vi "PPMSDR - Read lockin vs time_1.0.vi"(8 "stop":bool, 10 "Comments":string="Warmup\nVbg=0V\nVsg: NA\n\n200uV ac\nI+/I-: 2/5 200uVac\nI2+/-: 27/3 200uVac\nV+/V-: 3/27\nV3+/-: 4/28\nVsg: NA\n", 11 "folder name":string="monitor") -> (1 "X1":cluster{"Y":dbl[], "Y":dbl[]}[](graph), 3 "Temp vs Time":cluster{"Y":dbl[], "Y":dbl[]}[](graph), 5 "X4":cluster{"Y":dbl[], "Y":dbl[]}[](graph))   [LabVIEW 2013]
uses:
  <userlib>/Levylab/PPMS VI/Lock-in Globles.vi
  <userlib>/Levylab/PPMS VI/SubVI/ITX_Global.vi
  QDServer/QDServGlobal.vi
  <vilib>/Utility/file.llb/Write To Spreadsheet File (string).vi
panel:
  in  "Tab Control":T1(tab)
  in  "milliseconds to wait":u32=1000
  out "Connected":string="I-:4\nV2+:28\nI+:1\nV1+:2\nV-:3\nV2-:5\n"
  in  "Lockins":i32[](array[numeric])=[0, 1, 2, 3, 4, 5]
  out "Array X":dbl[](array[numeric])=[5.264924893925422e-11, 1.3604655963589375e-10, 5.1217581158894604e-08, 4.031695120308963e-16, -1.3552086788225654e-05, 3.1233416285824434e-11]
  out "Array Y":dbl[](array[numeric])=[-3.141694202030661e-12, -8.008054257042766e-12, -2.1068074715954563e-08, 8.074647968603996e-16, 1.39380477016865e-07, -2.3056960893811664e-13]
  in  "2 Frequencies?":bool
  out "X0":cluster{"Y":dbl[], "Y":dbl[]}[](graph)
  out "X2":cluster{"Y":dbl[], "Y":dbl[]}[](graph)
  out "X3":cluster{"Y":dbl[], "Y":dbl[]}[](graph)
  out "X5":cluster{"Y":dbl[], "Y":dbl[]}[](graph)
  out "R":cluster{"Y":dbl[], "Y":dbl[]}[](graph)
  in  "V1":i32
  in  "Current":i32=1
  in  "V2":i32
  out "B vs Time":cluster{"Y":dbl[], "Y":dbl[]}[](graph)
  out "R vs T":cluster{"Y":dbl[], "Y":dbl[]}[](graph)
  # "0,1,2,3 ect."
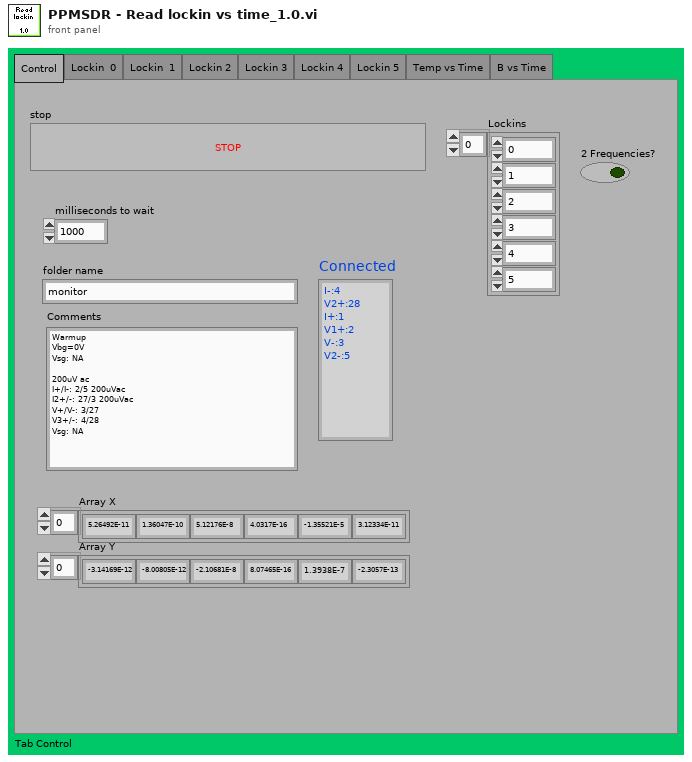
[diagram p1: front panel]
types:
  T1 = enum32{"Control", "Lockin  0", "Lockin  1", "Lockin 2", "Lockin 3", "Lockin 4", "Lockin 5", "Temp vs Time", "B vs Time"}
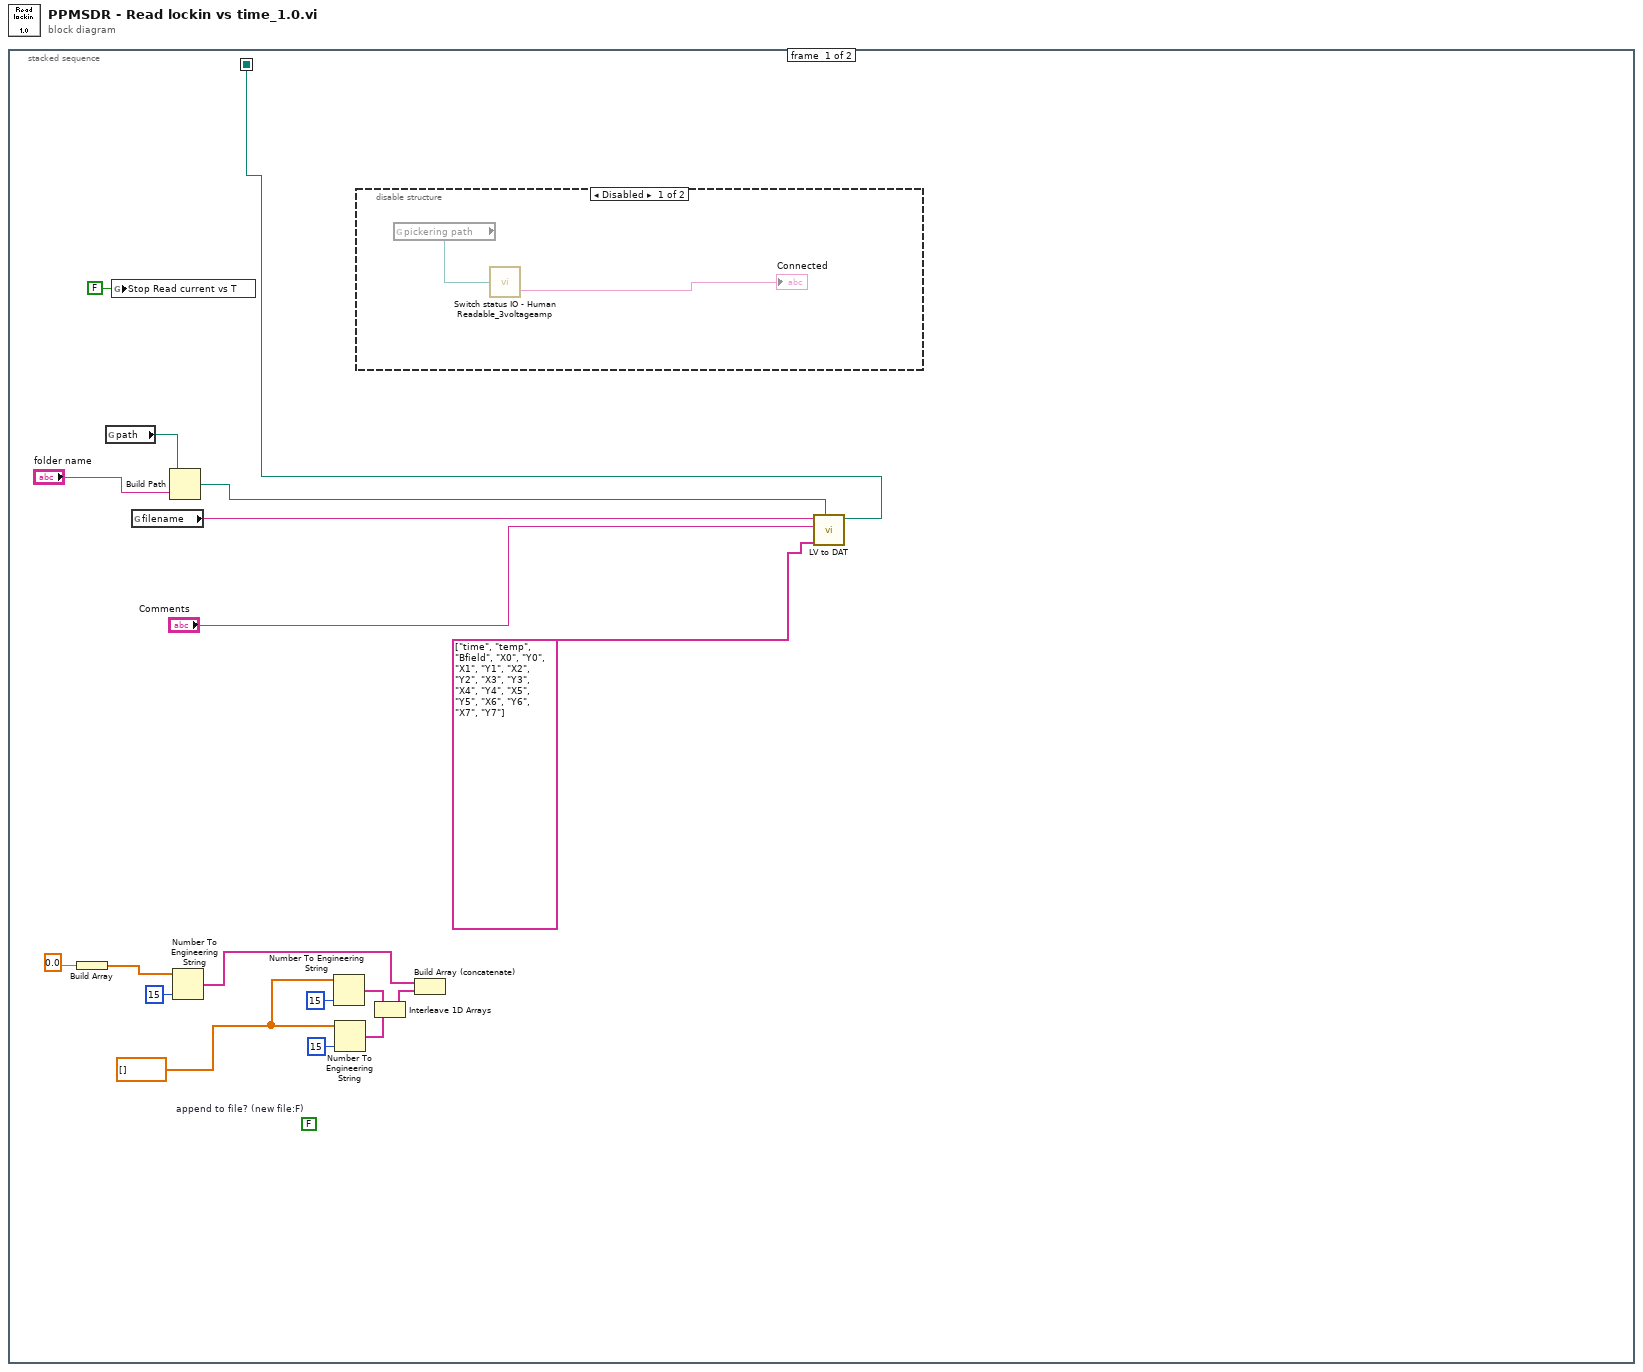
[diagram p0: block diagram]
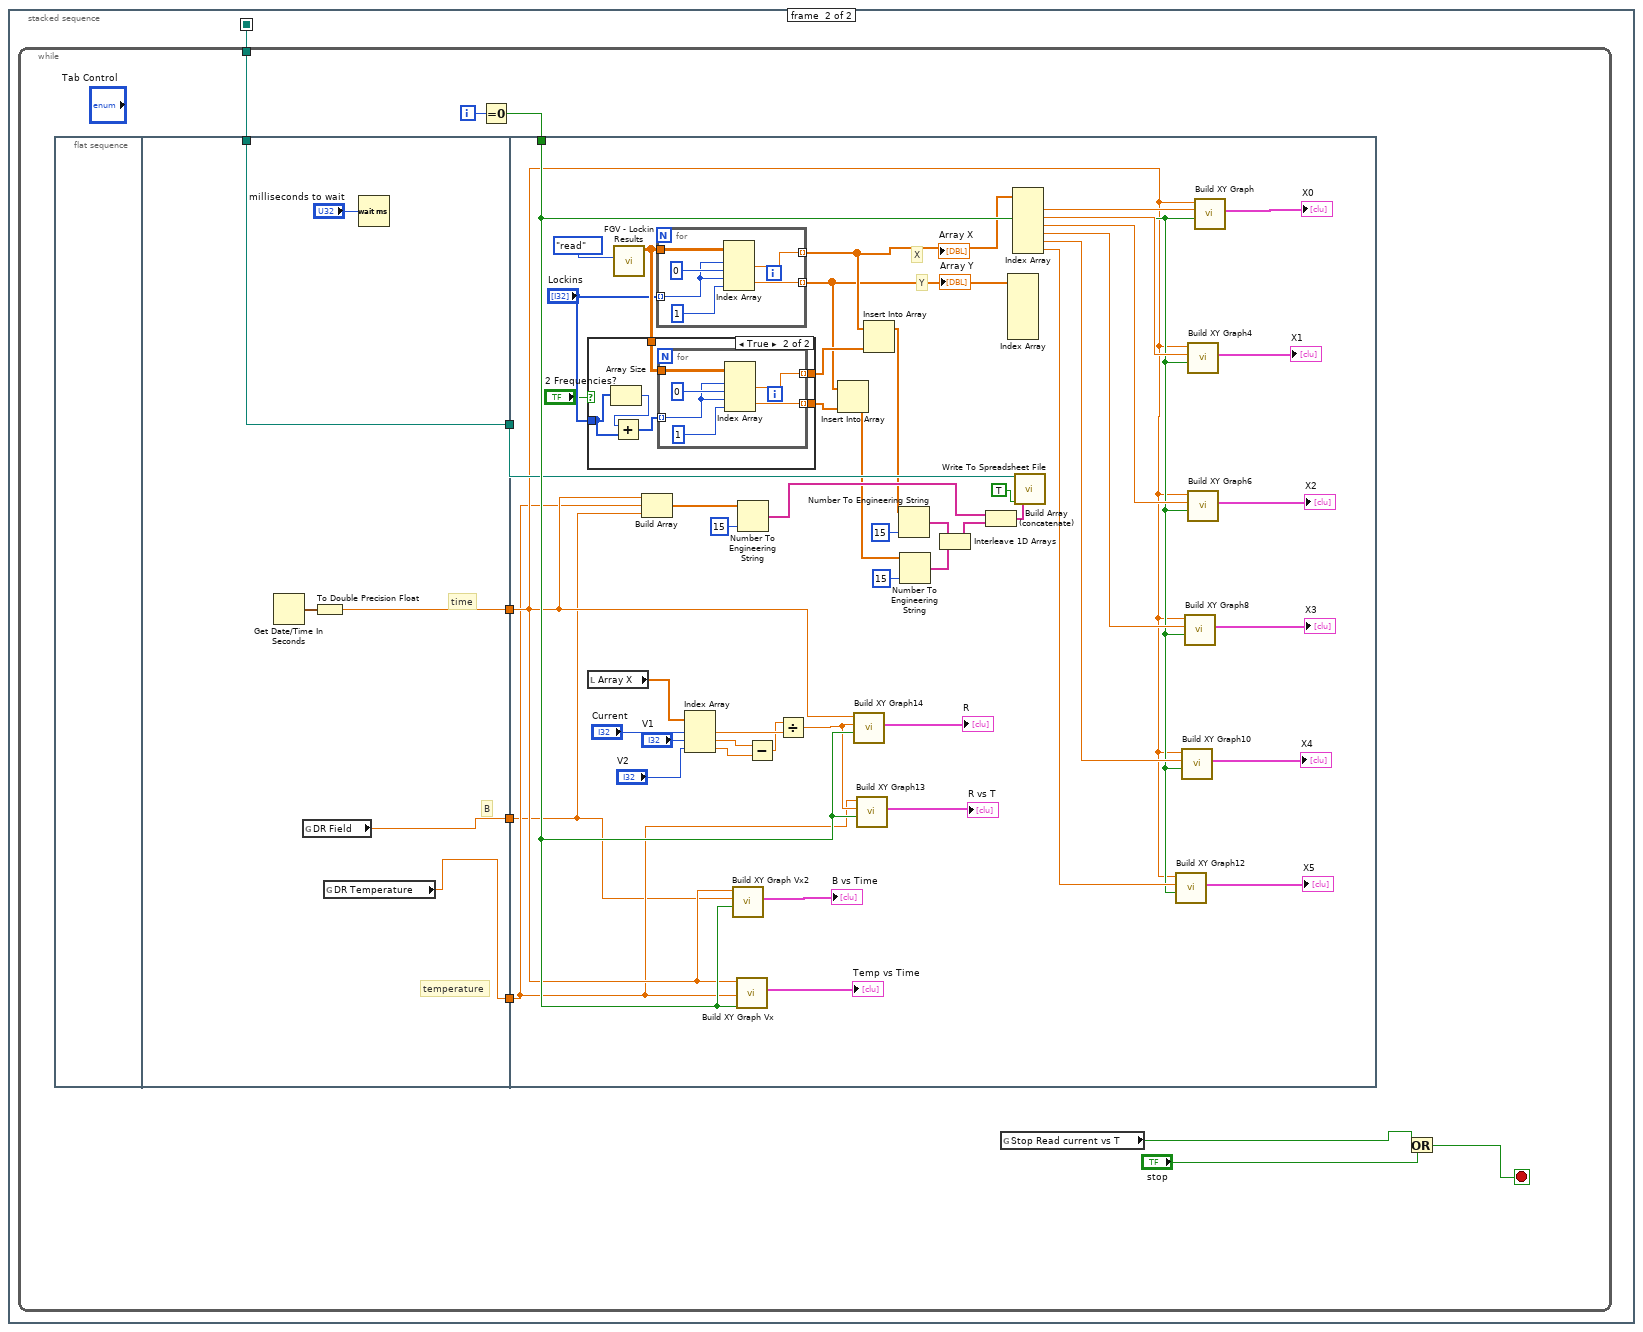
[diagram p3: hidden frame]
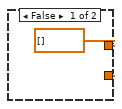
[diagram p4: hidden frame]
diagram:
  n1 = stacked-sequence {
    seq-local: [w1 _] -> [_ w21]
    frame #0 {
      w6 = dbl[] []
      (unwired) FALSE  # append to file? (new file:F)
      n2 = Build Array(0.0) -> (w12:dbl[])
      n3 = global read "ITX_Global.vi" "path"() -> (w17:path)
      n4 = global write "Lock-in Globles.vi" "Stop Read current vs T"(FALSE ("Stop Read current vs T")) -> ()
      n5 = global read "ITX_Global.vi" "filename"() -> (w3:string)
      n6 = Build Path(base path=w17, name or relative path="folder name") -> (appended path=w2:path)
      n7 = Number To Engineering String(2:i16 15 ("precision (6)"), 4:w12) -> (0:w11:string[])  [unwired: 2 out]
      n8 = Number To Engineering String(2:i16 15 ("precision (6)"), 4:w6) -> (0:w10:string[])  [unwired: 2 out]
      n9 = Number To Engineering String(2:i16 15 ("precision (6)"), 4:w6) -> (0:w9:string[])  [unwired: 2 out]
      n10 = disable-structure shown="Disabled" {
        frame Disabled {
          n11 = global read "ITX_Global.vi" "pickering path"() -> (w19:path)
          n12 = call <userlib>:"Switch status IO - Human Readable_3voltageamp.vi"("Switch status"=w19) -> ("String"=→"Connected":string)  [unwired: 3 in]
        }
        frame Enabled {
        }
      }
      n13 = Interleave 1D Arrays(w10, w9) -> (w8:string[])
      n14 = Build Array (concatenate)(w11, w8) -> ()  [unwired: 1 out]
      n15 = call <userlib>:"LV to DAT.vi"("path"=w2, "wavenames (.Vx, etc)"=string[] ["time", "temp", "Bfield", "X0", "Y0", "X1", "Y1", "X2", "Y2", "X3", "Y3", "X4", "Y4", "X5", "Y5", "X6", "Y6", "X7", "Y7"], "Comments"="Comments", "filename"=w3) -> ("new file path (Not A Path if cancelled)"=w1:path)  [unwired: 7 in]
    }
    frame #1 {
      n16 = while {
        tunnel: w21 -> [w24]
        i -> [w31]
        stop <- w25 stop-if-true
        n17 = flat-sequence {
          tunnel: [w35] -> w29
          tunnel: [w32] -> w27
          tunnel: [w33] -> w26
          tunnel: w24 -> [w34]
          tunnel: [w34] -> w23
          tunnel: w30 -> [w66]
          tunnel: w29 -> [w56]
          tunnel: w27 -> [w55]
          tunnel: w26 -> [w54]
          tunnel: w23 -> [w64]
          frame #0 {
          }
          frame #1 {
            # "B"
            # "time"
            # "temperature"
            n18 = Get Date/Time In Seconds() -> (seconds since 1Jan1904=w36:timestamp)
            n19 = global read "QDServGlobal.vi" "DR Field"() -> (w33:dbl)
            n20 = To Double Precision Float(number=w36) -> (double precision float=w35:dbl)
            n21 = global read "QDServGlobal.vi" "DR Temperature"() -> (w32:dbl)
            n22 = Wait (ms)(milliseconds to wait="milliseconds to wait") -> ()  [unwired: 1 out]
          }
          frame #2 {
            # "Y"
            # "X"
            n23 = local read "Array X"() -> (w61:dbl[])
            n24 = call <userlib>:"FGV - Lockin Results.vi"("Function"=enum16{"write", "read"}."read") -> ("Input Signals"=w46:dbl[][])  [unwired: 5 in, 1 out]
            n25 = case shown="True" "2 Frequencies?" {
              tunnel: w46 -> [_ w94]
              tunnel: "Lockins" -> [_ w92]
              tunnel: [w88 w90] -> w42
              tunnel: [w88 w89] -> w39
              frame False {
                w88 = dbl[] []
              }
              frame True {
                n26 = Array Size(array=w92) -> (size(s)=w93:i32)
                n27 = Add(x=w93, y=w92) -> (x+y=w91:i32[])
                n28 = for {
                  tunnel: w94 -> [w97]
                  tunnel: w91 -> [w98] mode=indexing
                  tunnel: [w95] -> w90 mode=indexing
                  tunnel: [w96] -> w89 mode=indexing
                  n29 = Index Array(array=w97, index (row) #1=w98, index (col) #1=0 ("disabled index (col)"), index (row) #2=w98, index (col) #2=1 ("disabled index (col)")) -> (element #1=w95:dbl, element #2=w96:dbl)
                }
              }
            }
            n30 = Build Array(w56, w55, w54) -> (w53:dbl[])
            n31 = for {
              tunnel: w46 -> [w103]
              tunnel: "Lockins" -> [w104] mode=indexing
              tunnel: [w101] -> w43 mode=indexing
              tunnel: [w102] -> w40 mode=indexing
              n32 = Index Array(array=w103, index (row) #1=w104, index (col) #1=0 ("disabled index (col)"), index (row) #2=w104, index (col) #2=1 ("disabled index (col)")) -> (element #1=w101:dbl, element #2=w102:dbl)
            }
            "Array X" <- w43
            "Array Y" <- w40
            n33 = Index Array(array=w61, index #1="Current", index #2="V1", index #3="V2") -> (element #1=w70:dbl, element #2=w60:dbl, element #3=w59:dbl)
            n34 = call "Build XY Graph Vx2"("Reset"=w66, "Y Input"=w54, "X Input"=w56) -> ("XY Graph"=→"B vs Time":cluster{"Y":dbl[], "Y":dbl[]}[])  [unwired: 2 in, 6 out]
            n35 = call "Build XY Graph Vx"("Reset"=w66, "Y Input"=w55, "X Input"=w56) -> ("XY Graph"=→"Temp vs Time":cluster{"Y":dbl[], "Y":dbl[]}[])  [unwired: 2 in, 6 out]
            n36 = Number To Engineering String(2:i16 15 ("precision (6)"), 4:w53) -> (0:w52:string[])  [unwired: 2 out]
            n37 = Subtract(x=w60, y=w59) -> (x-y=w62:dbl)
            n38 = Divide(x=w62, y=w70) -> (x/y=w63:dbl)
            n39 = Insert Into Array(array=w40, new element=w39) -> (w38:dbl[])  [unwired: 1 in]
            n40 = call "Build XY Graph14"("Reset"=w66, "Y Input"=w63, "X Input"=w56) -> ("XY Graph"=→"R":cluster{"Y":dbl[], "Y":dbl[]}[])  [unwired: 2 in, 6 out]
            n41 = call "Build XY Graph13"("Reset"=w66, "Y Input"=w63, "X Input"=w55) -> ("XY Graph"=→"R vs T":cluster{"Y":dbl[], "Y":dbl[]}[])  [unwired: 2 in, 6 out]
            n42 = Insert Into Array(array=w43, new element=w42) -> (w41:dbl[])  [unwired: 1 in]
            n43 = Number To Engineering String(2:i16 15 ("precision (6)"), 4:w41) -> (0:w49:string[])  [unwired: 2 out]
            n44 = Number To Engineering String(2:i16 15 ("precision (6)"), 4:w38) -> (0:w48:string[])  [unwired: 2 out]
            n45 = Interleave 1D Arrays(w49, w48) -> (w47:string[])
            n46 = Build Array (concatenate)(w52, w47) -> (w51:string[])
            n47 = Index Array(array=w40) -> ()  [unwired: 6 in, 6 out]
            n48 = Index Array(array=w43) -> (element #1=w86:dbl, element #2=w84:dbl, element #3=w82:dbl, element #4=w80:dbl, element #5=w78:dbl, element #6=w76:dbl)  [unwired: 6 in]
            n49 = call-poly <vilib>:"Write To Spreadsheet File.vi"("append to file? (new file:F)"=TRUE, "1D data"=w51, "file path (dialog if empty)"=w64) -> ()  [unwired: 5 in, 1 out]
            n50 = call "Build XY Graph12"("Reset"=w66, "Y Input"=w76, "X Input"=w56) -> ("XY Graph"=→"X5":cluster{"Y":dbl[], "Y":dbl[]}[])  [unwired: 2 in, 6 out]
            n51 = call "Build XY Graph10"("Reset"=w66, "Y Input"=w78, "X Input"=w56) -> ("XY Graph"=→"X4":cluster{"Y":dbl[], "Y":dbl[]}[])  [unwired: 2 in, 6 out]
            n52 = call "Build XY Graph8"("Reset"=w66, "Y Input"=w80, "X Input"=w56) -> ("XY Graph"=→"X3":cluster{"Y":dbl[], "Y":dbl[]}[])  [unwired: 2 in, 6 out]
            n53 = call "Build XY Graph4"("Reset"=w66, "Y Input"=w84, "X Input"=w56) -> ("XY Graph"=→"X1":cluster{"Y":dbl[], "Y":dbl[]}[])  [unwired: 2 in, 6 out]
            n54 = call "Build XY Graph6"("Reset"=w66, "Y Input"=w82, "X Input"=w56) -> ("XY Graph"=→"X2":cluster{"Y":dbl[], "Y":dbl[]}[])  [unwired: 2 in, 6 out]
            n55 = call "Build XY Graph"("Reset"=w66, "Y Input"=w86, "X Input"=w56) -> ("XY Graph"=→"X0":cluster{"Y":dbl[], "Y":dbl[]}[])  [unwired: 2 in, 6 out]
          }
        }
        n56 = Equal To 0?(x=w31) -> (x = 0?=w30:bool)
        n57 = global read "Lock-in Globles.vi" "Stop Read current vs T"() -> (w22:bool)
        n58 = Or(x=w22, y="stop") -> (x .or. y?=w25:bool)
      }
    }
  }
